vi "Relation Definition.vi"(11 "Relation in":refnum<class "Relation.lvclass">) -> (1 "Relation Definition":T1, 2 "Table Name":string, 3 "Relation out":refnum<class "Relation.lvclass">)   [LabVIEW 2020, in "Conditum.lvlib" / "Columns.lvlib" / "Relation.lvclass"]
uses:
  Relation.lvclass
  Relation.lvclass/Relation.ctl
  Type/Type.lvclass
  C:/dev/lv20CE/lv-conditum/Conditum/Columns/Type/Type.lvclass
  C:/dev/lv20CE/lv-conditum/Conditum/Columns/Relation/Relation.lvclass
  Relation Mapping.ctl
  Conditum.lvlib
  Relation Info.ctl
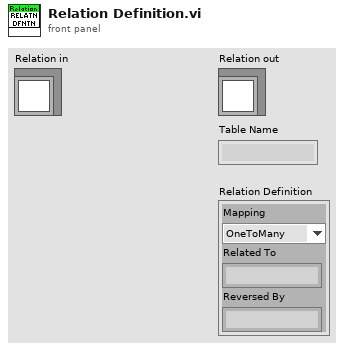
[diagram p1: front panel]
types:
  T1 = typedef "Conditum.lvlib/Relation Info.ctl" = cluster{"Mapping":T2, "Related To":string, "Reversed By":string}
  T2 = typedef "Conditum.lvlib/Relation Mapping.ctl" = enum16{"OneToMany", "ManyToOne", "ManyToMany", "OneToOne"}
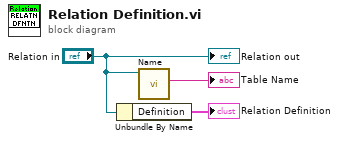
[diagram p0: block diagram]
diagram:
  n1 = Unbundle By Name("Relation in") -> ("Definition"=→"Relation Definition":T1)
  n2 = call "Name.vi"("Type in"="Relation in") -> ("Table Name"=→"Table Name":string)  [unwired: 10 in]
  "Relation out" <- "Relation in"
